vi "Configure Output.vi"(8 "error in (no error)":errorcluster, 10 "Output Setting":T1, 11 "BK-Precision in":refnum<class "BK-Precision.lvclass">) -> (0 "error out":errorcluster, 3 "BK-Precision out":refnum<class "BK-Precision.lvclass">)   [LabVIEW 2016, in "DC PWS.lvlib" / "BK-Precision.lvclass"]
uses:
  BK-Precision.lvclass
  BK-Precision.lvclass/BK-Precision.ctl
  <instrlib>/BK Precision 911X Series/BK Precision 911X Series.lvlib
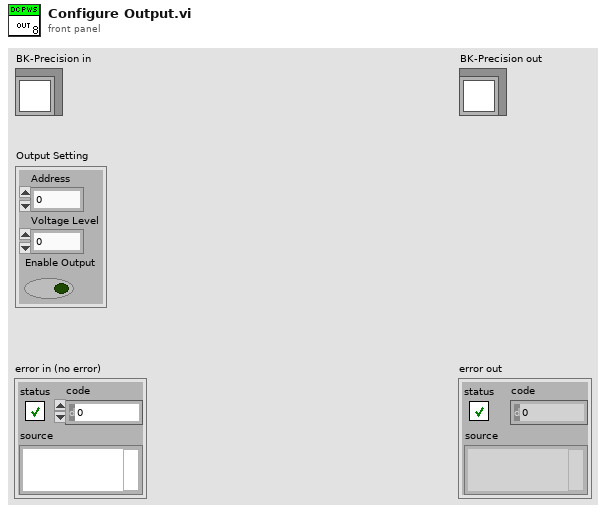
[diagram p1: front panel]
types:
  T1 = cluster{"Address":dbl, "Voltage Level":dbl, "Enable Output":bool}
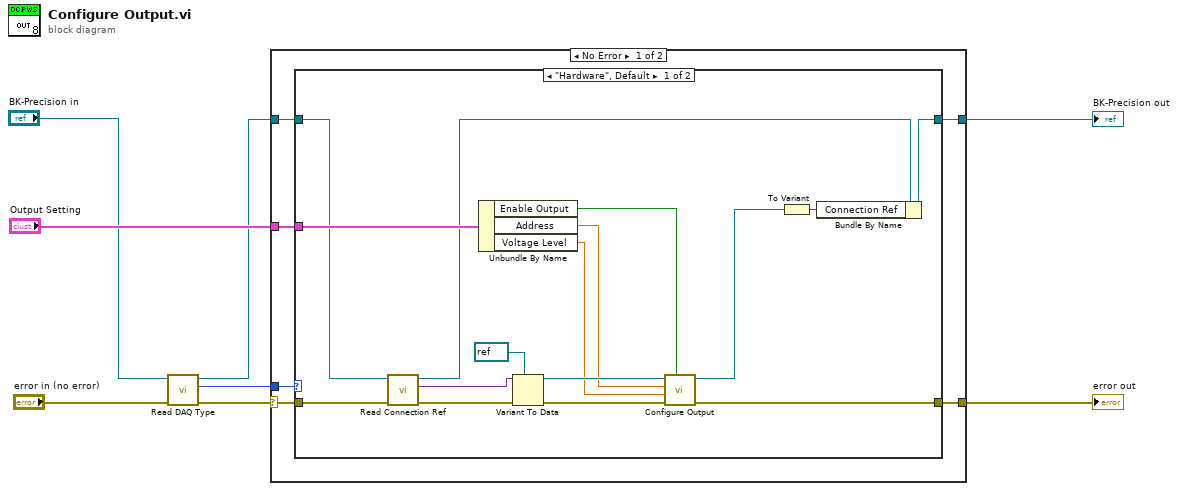
[diagram p0: block diagram]
diagram:
  n1 = call "Read DAQ Type.vi"("error in (no error)"="error in (no error)", "BK-Precision in"="BK-Precision in") -> ("error out"=w7:errorcluster, "Type"=w6:enum16{"Hardware", "Simulation"}, "BK-Precision out"=w1:refnum<class "BK-Precision.lvclass">)  [unwired: 7 in]
  n2 = case shown="No Error" w7 {
    selector: w7 -> [w13 w33]
    tunnel: w6 -> [w14 _]
    tunnel: w1 -> [w12 w34]
    tunnel: [w11 w34] -> w5
    tunnel: [w10 w33] -> w4
    tunnel: "Output Setting" -> [w9 _]
    frame No Error {
      n3 = case shown="\"Hardware\", Default" w14 {
        tunnel: w13 -> [w30 w31]
        tunnel: w12 -> [w16 w32]
        tunnel: [w24 w32] -> w11
        tunnel: [w22 w31] -> w10
        tunnel: w9 -> [w21 _]
        frame "Hardware", Default {
          n4 = call "Read Connection Ref.vi"("error in (no error)"=w30, "BK-Precision in"=w16) -> ("error out"=w29:errorcluster, "Conn Ref"=w28:variant, "BK-Precision out"=w15:refnum<class "BK-Precision.lvclass">)  [unwired: 7 in]
          n5 = Unbundle By Name(w21) -> ("Enable Output"=w18:bool, "Address"=w20:dbl, "Voltage Level"=w19:dbl)
          n6 = Variant To Data(error in=w29, type=refnum<visa-resource-name> refnum ("VISA resource name"), Variant=w28) -> (data=w25:refnum<visa-resource-name>, error out=w26:errorcluster)
          n7 = call <instrlib>:"Configure Output.vi"("Enable Output (T: Enable)"=w18, "error in (no error)"=w26, "Voltage Level (0.0 V)"=w19, "Address (0)"=w20, "VISA resource name"=w25) -> ("error out"=w22:errorcluster, "VISA resource name out"=w23:refnum<visa-resource-name>)  [unwired: 5 in]
          n8 = To Variant(anything=w23) -> (Variant=w17:variant)
          n9 = Bundle By Name(cluster=w15, "Connection Ref"=w17) -> (w24:refnum<class "BK-Precision.lvclass">)
        }
        frame "Simulation" {
        }
      }
    }
    frame Error {
    }
  }
  "error out" <- w4
  "BK-Precision out" <- w5
